vi "White Balance.vi"(0 "wRed":u16, 1 "fRelB":sgl, 5 "wGreen":u16, 7 "wBlue":u16, 9 "fRelR":sgl, 12 "info":T1) -> (2 "function return":u32, 3 "fRelB out":sgl, 4 "wRed out":u16, 6 "wGreen out":u16, 8 "wBlue out":u16, 10 "fRelR out":sgl, 14 "info out":T1)   [LabVIEW 2018, in "Copy of Andor SDK.lvlib"]
doc: "EXPNETTYPE unsigned int WINAPI WhiteBalance(WORD * wRed, WORD * wGreen, WORD * wBlue, float * fRelR, float * fRelB, WhiteBalanceInfo * info);"
uses:
  Copy of Andor SDK.lvlib
  <userlib>/Andor SDK/ATMCD32D.dll
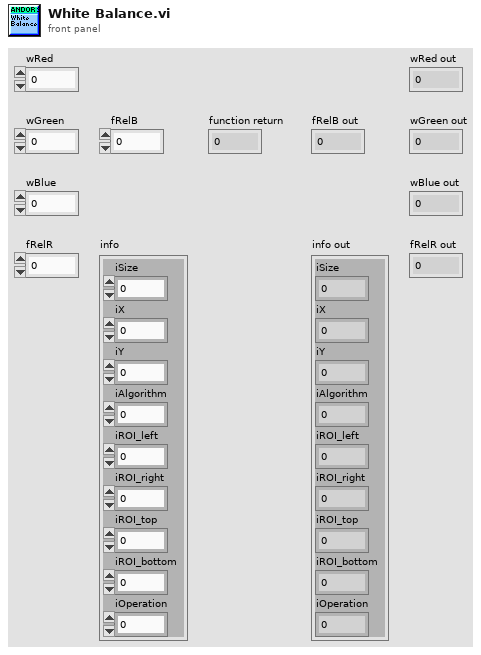
[diagram p1: front panel]
types:
  T1 = cluster{"iSize":i32, "iX":i32, "iY":i32, "iAlgorithm":i32, "iROI_left":i32, "iROI_right":i32, "iROI_top":i32, "iROI_bottom":i32, "iOperation":i32}
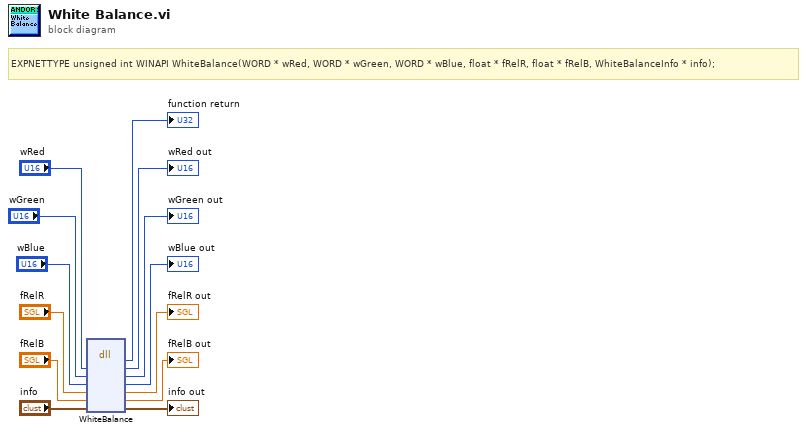
[diagram p0: block diagram]
diagram:
  # "EXPNETTYPE unsigned int WINAPI WhiteBalance(WORD * wRed, WORD * wGreen, WORD * wBlue, float * fRelR, float * fRelB, WhiteBalanceInfo * info);"
  n1 = dll-call lib="C:/Program Files (x86)/National Instruments/LabVIEW 2018/user.lib/Andor SDK/ATMCD32D.*" fn="WhiteBalance"("wRed"="wRed", "wGreen"="wGreen", "wBlue"="wBlue", "fRelR"="fRelR", "fRelB"="fRelB", "info"="info") -> (→"function return":u32, "wRed"=→"wRed out":u16, "wGreen"=→"wGreen out":u16, "wBlue"=→"wBlue out":u16, "fRelR"=→"fRelR out":sgl, "fRelB"=→"fRelB out":sgl, "info"=→"info out":T1)  [unwired: 3 in, 2 out]
